vi "Edit All Status Indicators.vi"(0 "Instrument Status Ouside":refnum<vi>, 1 "Instrument Status Inside":refnum<vi>, 3 "Error In":errorcluster, 4 "State":T1=enum."Moving") -> (10 "Error Out":errorcluster)   [LabVIEW 2014]
uses:
  Instrument Status.ctl
  Instrument Status State.ctl
panel:
  # "LICENSED MATERIALS – PROPERTY OF IBM\nCopyright IBM Corp. 2016, 2016\nALL RIGHTS RESERVED"
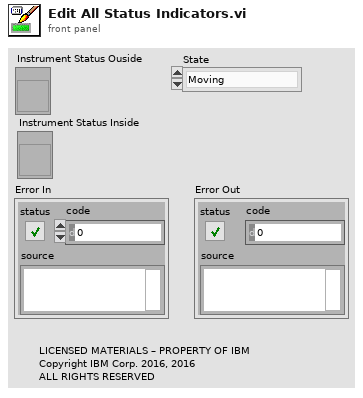
[diagram p1: front panel]
types:
  T1 = typedef "Instrument Status State.ctl" = enum16{"Unknown", "Idle", "Standby", "Configuring", "Measuring", "Moving", "Disconnected"}
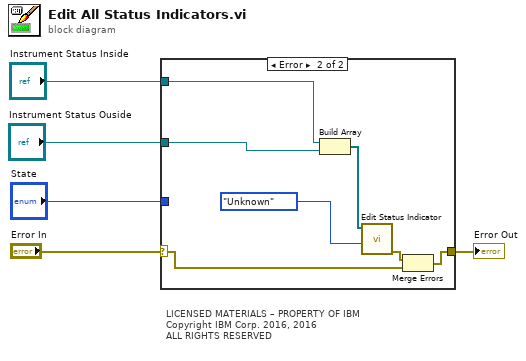
[diagram p0: block diagram]
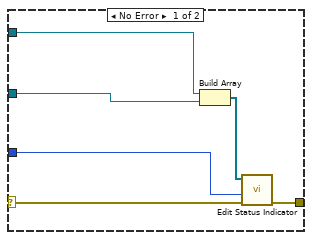
[diagram p2: hidden frame]
diagram:
  # "LICENSED MATERIALS – PROPERTY OF IBM\nCopyright IBM Corp. 2016, 2016\nALL RIGHTS RESERVED"
  n1 = case shown="Error" "Error In" {
    selector: "Error In" -> [w11 w17]
    tunnel: [w10 w16] -> w2
    tunnel: "Instrument Status Inside" -> [w8 w13]
    tunnel: "Instrument Status Ouside" -> [w7 w12]
    tunnel: "State" -> [w6 _]
    frame No Error {
      n2 = Build Array(w8, w7) -> (w9:refnum<vi>[])
      n3 = call "Edit Status Indicator.vi"("error in (no error)"=w11, "State"=w6, "Instrument Status Refnum"=w9) -> ("error out"=w10:errorcluster)  [unwired: 1 in, 7 out]
    }
    frame Error {
      n4 = Build Array(w13, w12) -> (w14:refnum<vi>[])
      n5 = call "Edit Status Indicator.vi"("State"=Instrument_Status_State."Unknown", "Instrument Status Refnum"=w14) -> ("error out"=w15:errorcluster)  [unwired: 2 in, 7 out]
      n6 = Merge Errors(w15, w17) -> (w16:errorcluster)
    }
  }
  "Error Out" <- w2
